vi "PRBS Mismatch Counter.vi"(7 "reset mismatch count":bool, 9 "input valid":bool, 10 "tkeep":bool[](array[boolean])=[FALSE, FALSE, FALSE, FALSE, FALSE, FALSE, FALSE, FALSE, FALSE, FALSE, FALSE, FALSE, FALSE, FALSE, FALSE, FALSE, FALSE, FALSE, FALSE, FALSE, FALSE, FALSE, FALSE, FALSE, FALSE, FALSE, FALSE, FALSE, FALSE, FALSE, FALSE, FALSE, FALSE, FALSE, FALSE, FALSE, FALSE, FALSE, FALSE, FALSE, FALSE, FALSE, FALSE, FALSE, FALSE, FALSE, FALSE, FALSE, FALSE, FALSE, FALSE, FALSE, FALSE, FALSE, FALSE, FALSE, FALSE, FALSE, FALSE, FALSE, FALSE, FALSE, FALSE, FALSE], 11 "data in":bool[](array[boolean])) -> (3 "mismatch count":u64)   [LabVIEW 2023, in "Aurora64b66b Utilities FPGA.lvlib"]
uses:
  Aurora64b66b Utilities FPGA.lvlib
  Program Files/NI/LVAddons/niidl/1/instr.lib/_niInstr/Data Formatting/v1/FPGA/niInstr Data Formatting v1 FPGA.lvlib
  Program Files/NI/LVAddons/niidl/1/instr.lib/_niInstr/Data Formatting/v1/FPGA/Private/Convert/Boolean Array to U64 Array.vi
  Program Files/NI/LVAddons/niidl/1/instr.lib/_niInstr/Basic Elements/v1/FPGA/niInstr Basic Elements v1 FPGA.lvlib
  Program Files/NI/LVAddons/niidl/1/instr.lib/_niInstr/Basic Elements/v1/FPGA/Private/Count Up U64.vi
  SubVIs/PRBS64 Parallel Rx - 4 Lanes.vi
  SubVIs/PRBS64 Parallel Rx - 8 Lanes.vi
  SubVIs/PRBS64 Parallel Rx - 16 Lanes.vi
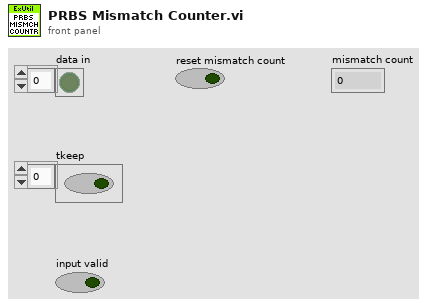
[diagram p1: front panel]
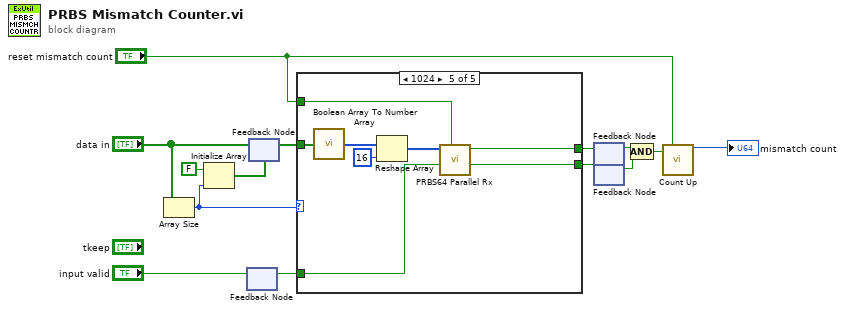
[diagram p0: block diagram]
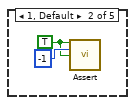
[diagram p3: hidden frame]
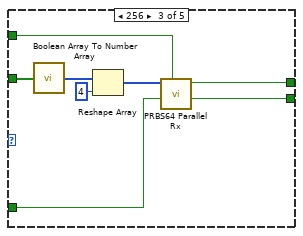
[diagram p4: hidden frame]
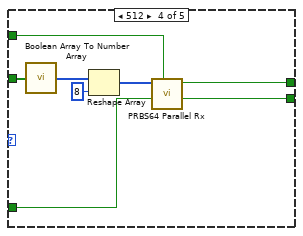
[diagram p5: hidden frame]
diagram:
  n1 = Array Size(array="data in") -> (size(s)=w8:i32)
  n2 = Initialize Array(FALSE, w8) -> (w13:bool[])
  n3 = feedback #1() -> (w9:bool)  [unwired: 1 in]
  n4 = feedback-in #1("input valid") -> ()
  n5 = feedback #2(w13) -> (w11:bool[])
  n6 = feedback-in #2("data in") -> ()
  n7 = case shown="1024" w8 {
    tunnel: w11 -> [_ _ w24 w32 w40]
    tunnel: "reset mismatch count" -> [_ _ w20 w27 w35]
    tunnel: [_ _ w18 w26 w34] -> w7
    tunnel: w9 -> [_ _ w19 w28 w36]
    tunnel: [_ _ w17 w25 w33] -> w3
    frame 0 {
    }
    frame 1, Default {
      w15 = TRUE ("assert")
      n8 = call "Assert.vi"("assert"=w15, "error code"=-1, "enable show error"=w15) -> ()  [unwired: 13 in]
    }
    frame 256 {
      n9 = call-poly "Boolean Array To Number Array.vi"("data in"=w24) -> ("data out"=w23:u64[])  [unwired: 14 in]
      n10 = Reshape Array(w23, 4 ("dimension size")) -> (w21:u64[])
      n11 = call-poly "PRBS64 Parallel Rx.vi"("reset"=w20, "input valid"=w19, "rx prbs"=w21) -> ("output valid"=w17:bool, "pattern mismatch"=w18:bool)  [unwired: 7 in]
    }
    frame 512 {
      n12 = call-poly "Boolean Array To Number Array.vi"("data in"=w32) -> ("data out"=w30:u64[])  [unwired: 14 in]
      n13 = Reshape Array(w30, 8 ("dimension size")) -> (w29:u64[])
      n14 = call-poly "PRBS64 Parallel Rx.vi"("reset"=w27, "input valid"=w28, "rx prbs"=w29) -> ("output valid"=w25:bool, "pattern mismatch"=w26:bool)  [unwired: 7 in]
    }
    frame 1024 {
      n15 = call-poly "Boolean Array To Number Array.vi"("data in"=w40) -> ("data out"=w38:u64[])  [unwired: 14 in]
      n16 = Reshape Array(w38, 16 ("dimension size")) -> (w37:u64[])
      n17 = call-poly "PRBS64 Parallel Rx.vi"("reset"=w35, "input valid"=w36, "rx prbs"=w37) -> ("output valid"=w33:bool, "pattern mismatch"=w34:bool)  [unwired: 7 in]
    }
  }
  n18 = feedback-in #3(w7) -> ()
  n19 = feedback #3() -> (w4:bool)  [unwired: 1 in]
  n20 = feedback #4() -> (w1:bool)  [unwired: 1 in]
  n21 = feedback-in #4(w3) -> ()
  n22 = Compound Arithmetic op=AND(w4, w1) -> (w2:bool)
  n23 = call-poly "Count Up.vi"("increment"=w2, "reset"="reset mismatch count") -> ("count out"=→"mismatch count":u64)  [unwired: 13 in]
